vi "constant--blank_core_data.vi"() -> (0 "blank core_data":T1)   [LabVIEW 2020, in "core.lvlib" / "core_data.lvlib"]
uses:
  core_data.lvlib
  core_data.ctl
  tour_in_progress.ctl
  chessboard_index.ctl
  chess_square.ctl
  neighbour_square.ctl
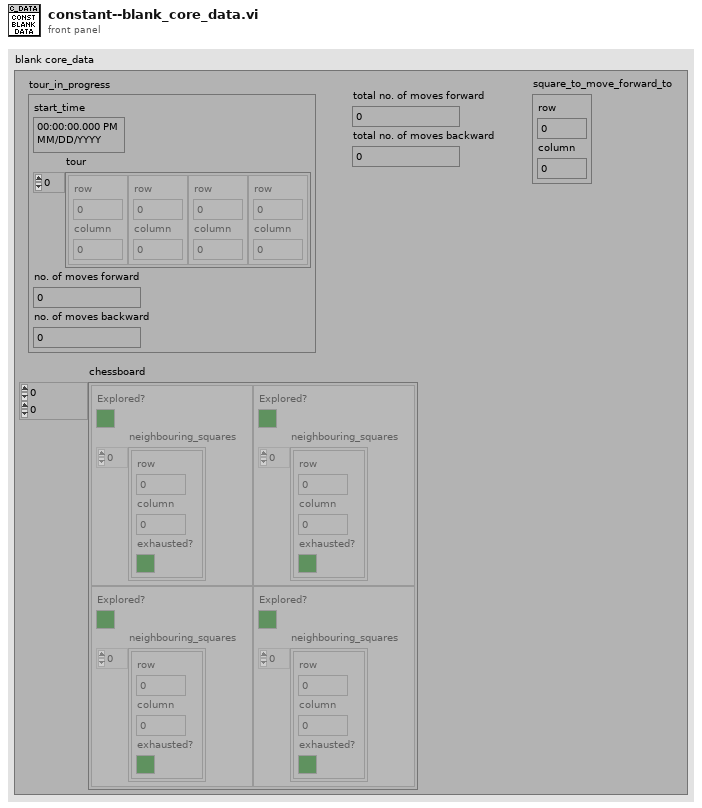
[diagram p1: front panel]
types:
  T1 = typedef "core.lvlib/core_data.lvlib/core_data.ctl" = cluster{"tour_in_progress":T2, "total no. of moves forward":u64, "total no. of moves backward":u64, "chessboard":T4[][], "square_to_move_forward_to":T3}
  T2 = typedef "core.lvlib/core_data.lvlib/tour_in_progress.ctl" = cluster{"start_time":timestamp, "tour":T3[], "no. of moves forward":u64, "no. of moves backward":u64}
  T3 = typedef "core.lvlib/core_data.lvlib/chessboard_index.ctl" = cluster{"row":u8, "column":u8}
  T4 = typedef "core.lvlib/core_data.lvlib/chess_square.ctl" = cluster{"Explored?":bool, "neighbouring_squares":T5[]}
  T5 = typedef "core.lvlib/core_data.lvlib/neighbour_square.ctl" = cluster{"row":u8, "column":u8, "exhausted?":bool}
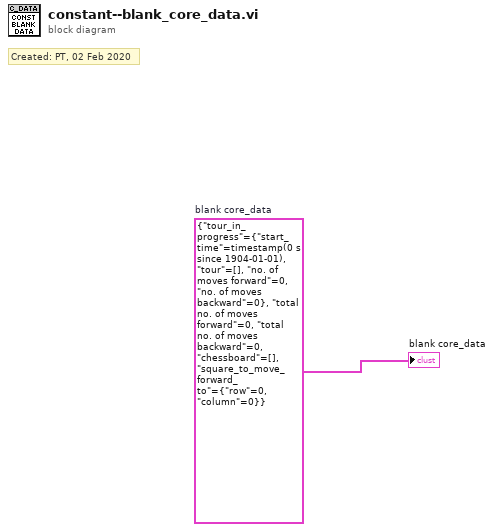
[diagram p0: block diagram]
diagram:
  w1 = T1 {"tour_in_progress"={"start_time"=timestamp(0 s since 1904-01-01), "tour"=[], "no. of moves forward"=0, "no. of moves backward"=0}, "total no. of moves forward"=0, "total no. of moves backward"=0, "chessboard"=[], "square_to_move_forward_to"={"row"=0, "column"=0}}  # blank core_data
  # "Created: PT, 02 Feb 2020"
  "blank core_data" <- w1
